vi "通讯测试.vi"() -> ()   [LabVIEW 2020]
panel:
  out "软件版本指示":T1 items=["for 广汽新能源"=24004, "for 中航锂电"=25006, ""=0]
  out "占空比判定":bool
  out "频率判定":bool
  out "软件版本号":u32
  out "?":bool
  out "表格控件":string[][](table) caption="温度通讯结果"
  out "频率/周期":u32
  out "占空比":u32
  out "error out":errorcluster caption="错误输出"
  in  "error in":errorcluster caption="错误输入"
  # "F020  通讯测试"
  # "HVIL测试"
  # "Hz"
  # "判定：10±1Hz"
  # "判定：50±5%"
  # "%"
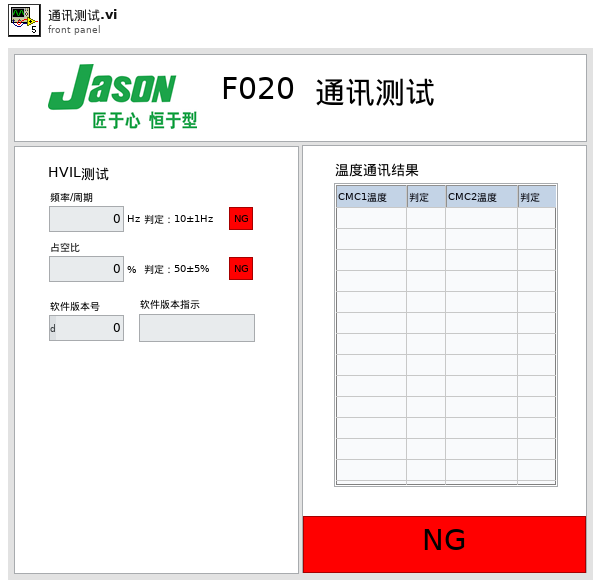
[diagram p1: front panel]
types:
  T1 = typedef "软件版本指示.ctl" = u32
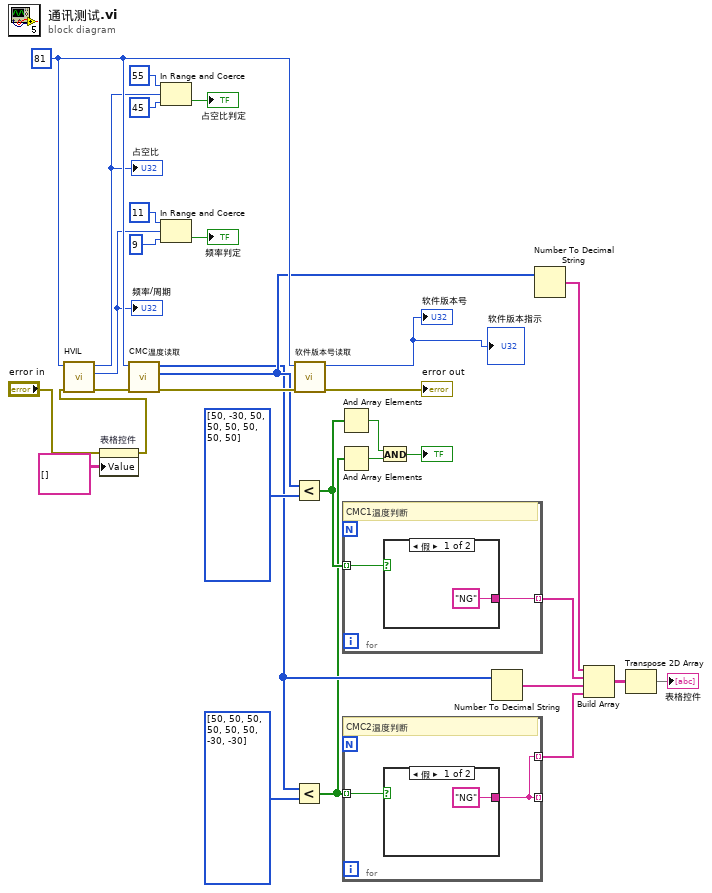
[diagram p0: block diagram]
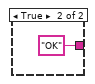
[diagram p2: hidden frame]
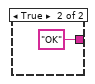
[diagram p3: hidden frame]
diagram:
  w29 = u16 81 ("Channel")
  n1 = property on="表格控件" class="Tbl (严格)"(error in="error in", "Value"=string[][] [] ("表格控件")) -> (error out=w2:errorcluster)  [unwired: 1 in, 1 out]
  n2 = call "HVIL.vi"("error in"=w2, "Channel"=w29) -> ("error out"=w13:errorcluster, "频率/周期"=w12:u32, "占空比"=w8:u32)  [unwired: 7 in]
  "占空比" <- w8
  "频率/周期" <- w12
  n3 = call "CMC温度读取.vi"("error in"=w13, "Channel"=w29) -> ("error out"=w31:errorcluster, "CMC1温度"=w26:i32[], "CMC2温度"=w25:i32[])  [unwired: 7 in]
  n4 = In Range and Coerce(upper limit=u32 55 ("上限"), x=w8, lower limit=u32 45 ("下限")) -> (In Range?=→"占空比判定":bool)  [unwired: 1 out]
  n5 = In Range and Coerce(upper limit=u32 11 ("上限"), x=w12, lower limit=u32 9 ("下限")) -> (In Range?=→"频率判定":bool)  [unwired: 1 out]
  n6 = Less?(x=w26, y=i32[] [50, -30, 50, 50, 50, 50, 50, 50]) -> (x < y?=w18:bool[])
  n7 = Less?(x=w25, y=i32[] [50, 50, 50, 50, 50, 50, -30, -30]) -> (x < y?=w17:bool[])
  n8 = call "软件版本号读取.vi"("error in"=w31, "Channel"=w29) -> ("error out"=→"error out":errorcluster, "软件版本号"=→"软件版本号" →"软件版本指示":u32)  [unwired: 8 in]
  n9 = And Array Elements(Boolean array=w18) -> (logical AND=w16:bool)
  n10 = And Array Elements(Boolean array=w17) -> (logical AND=w15:bool)
  n11 = for {
    tunnel: w18 -> [w33] mode=indexing
    tunnel: [w32] -> w23 mode=indexing
    # "CMC1温度判断"
    n12 = case shown="假" w33 {
      tunnel: ["NG" "OK"] -> w32
      frame False {
      }
      frame True {
      }
    }
  }
  n13 = for {
    tunnel: w17 -> [w37] mode=indexing
    tunnel: [w36] -> _ mode=indexing
    tunnel: [w36] -> w21 mode=indexing
    # "CMC2温度判断"
    n14 = case shown="假" w37 {
      tunnel: ["NG" "OK"] -> w36
      frame False {
      }
      frame True {
      }
    }
  }
  n15 = And(x=w16, y=w15) -> (x .and. y?=→"?":bool)
  n16 = Number To Decimal String(number=w25) -> (decimal integer string=w22:string[])  [unwired: 1 in]
  n17 = Number To Decimal String(number=w26) -> (decimal integer string=w24:string[])  [unwired: 1 in]
  n18 = Build Array(w24, w23, w22, w21) -> (w20:string[][])
  n19 = Transpose 2D Array(2D array=w20) -> (transposed array=→"表格控件":string[][])
